vi "1_VNA_direct_spectrum_field_sweep_CURRENT_(2D_PNA_m_Field_Direct_spec_RHUL).vi"() -> ()   [LabVIEW 2013]
uses:
  <vilib>/Analysis/baseanly.llb/Mean (DBL).vi
  <vilib>/Analysis/NI_AALBase.lvlib
panel:
  in  "?":enum32{"Magnetic Field", "Cycle wait"}(tab)
  in  "I_start (mA)":dbl=-10.0 format="%#.3f"
  in  "I_end(mA)":dbl=6953330000.0 caption="Center Freq (Hz):" format="%#.6p"
  in  "n_points":i32=1000
  in  "Current":bool
  out "I current":dbl=3.2196
  in  "Cycle delay (s)":dbl
  in  "First step delay (s)":dbl
  in  "?":enum32{"VNA"}(tab)
  out "Numeric":i32
  in  "No averages":i32=3 caption="Delay Time (s)"
  in  "Background remove":bool
  in  "?":enum32{"VNA"}(tab)
  in  "VNA Power dBm":dbl=-30.0 caption="VNA Power (dBm)" format="%#.3f"
  in  "Center Freq (Hz)":dbl=9000000000.0 caption="Center Freq (Hz):" format="%#.6p"
  in  "Span Freq:":dbl=14000000000.0 caption="Span Freq (Hz)" format="%#.3p"
  in  "Bandwidth:":dbl=10.0 caption="Bandwidth (1 to 1e6 Hz)" format="%#.3f"
  in  "Points:":i32=201 caption="Points"
  out "Phase (now)":dbl[](graph)
  out "Amplitude (now)":dbl[](graph)
  in  "Phase delay (ns)":dbl=53.6 format="%#_8g"
  in  "Offset (rad)":dbl
  out "Phase Background Corrected":dbl[][](graph)
  out "Amplitude Background Corrected":dbl[][](graph)
  out "Phase Raw":dbl[][](graph)
  out "Amplitude Raw":dbl[][](graph)
  out "XY Graph":cluster{dbl[], dbl[]}(graph)
  out "Temp_start":dbl=2.0 format="%#_13g"
  out "Temp_end":dbl=16.0 format="%#_13g"
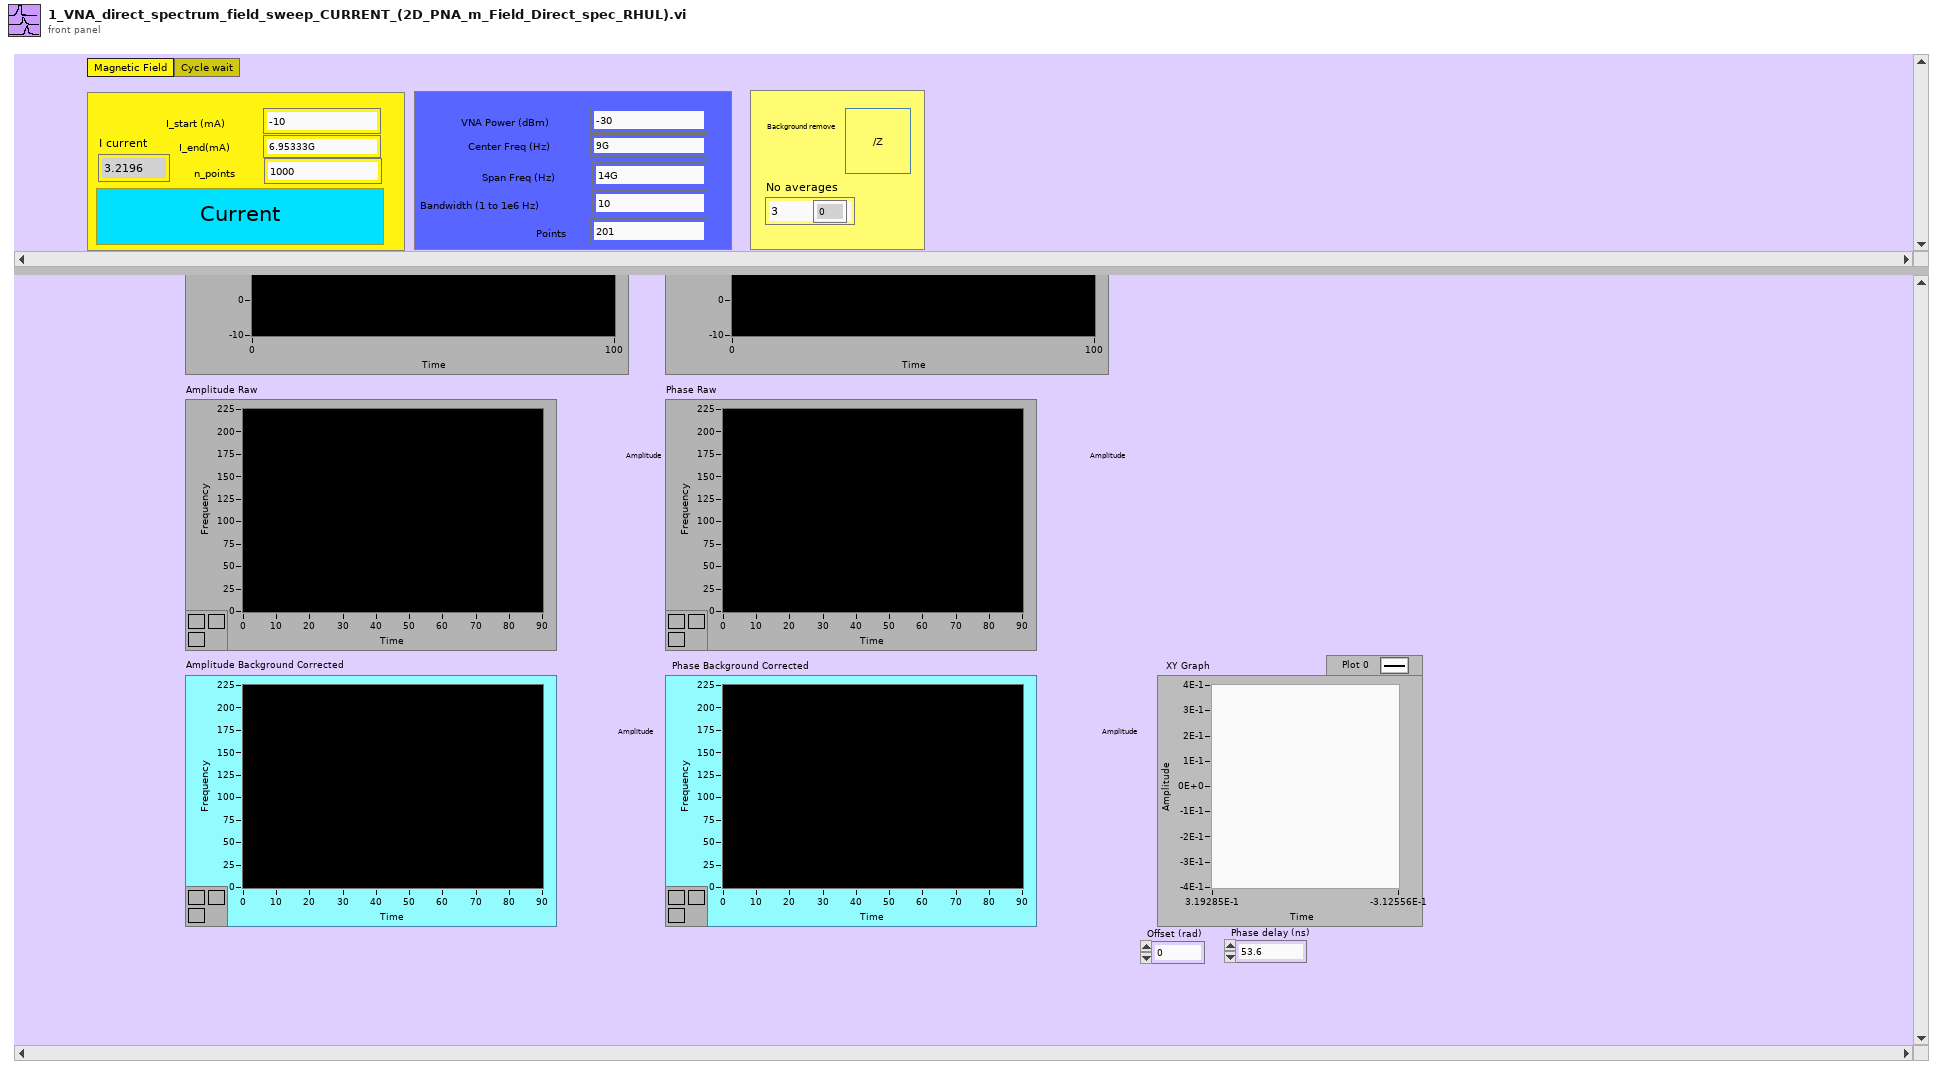
[diagram p1: front panel]
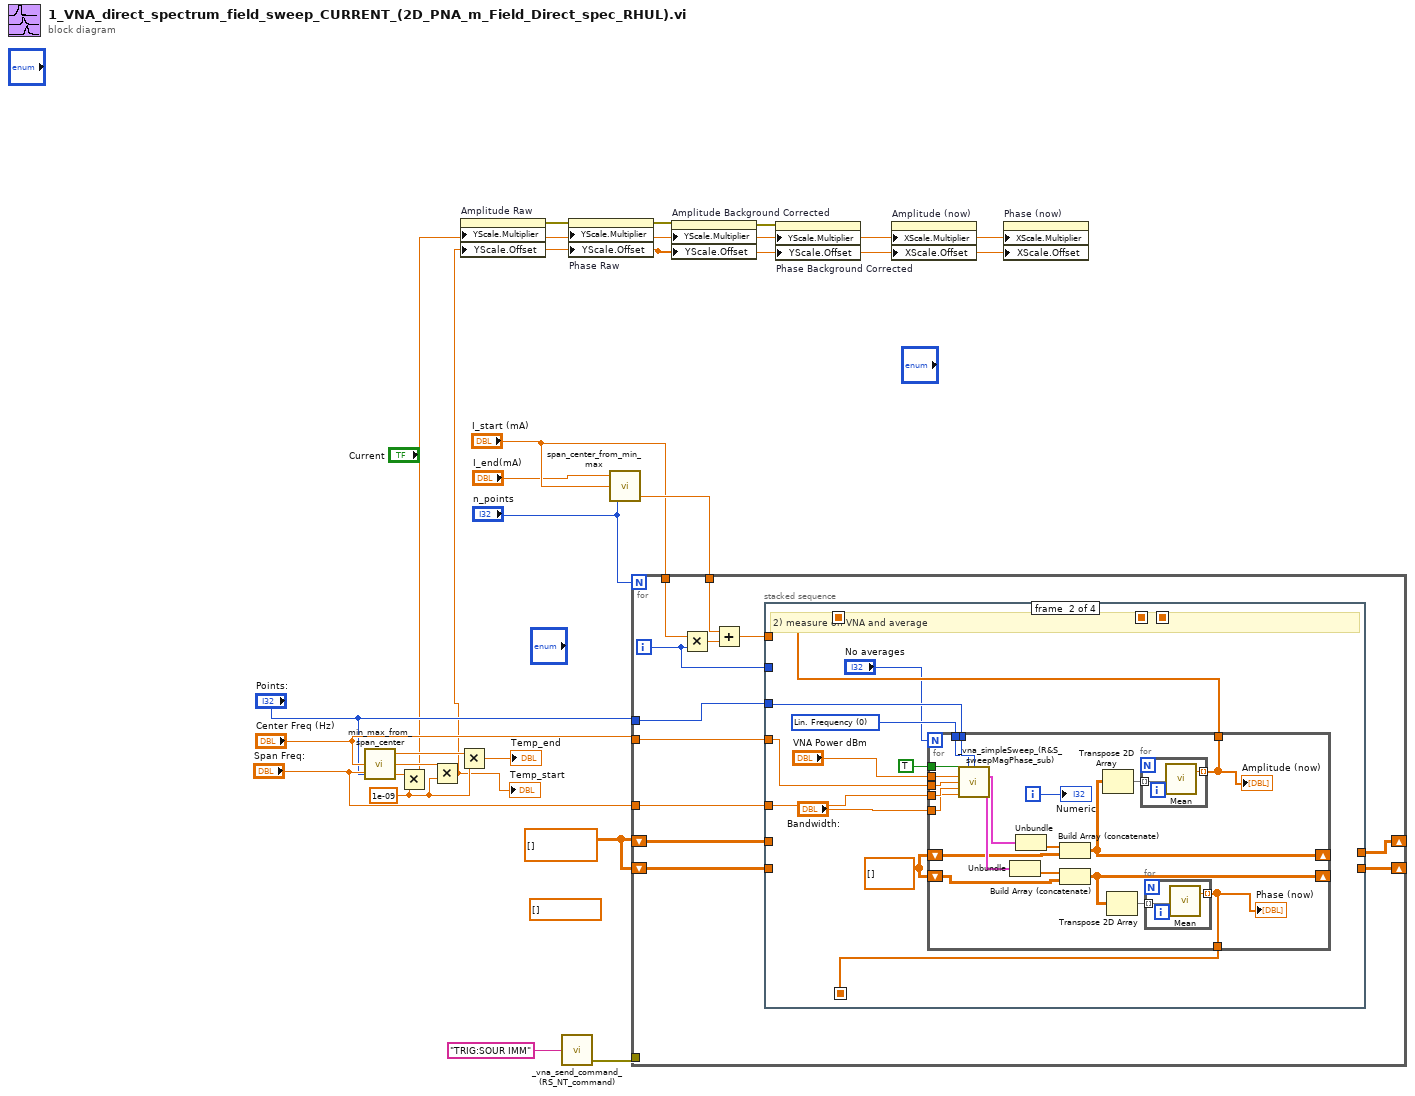
[diagram p0: block diagram]
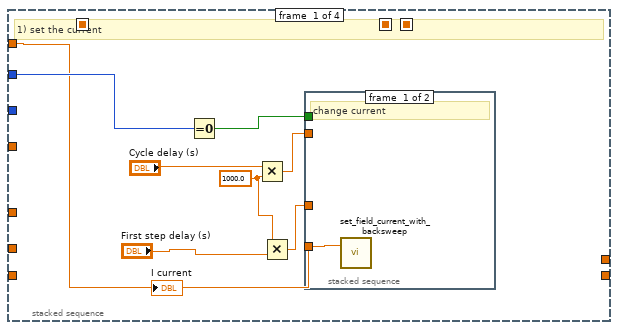
[diagram p2: hidden frame]
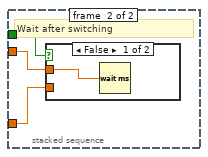
[diagram p3: hidden frame]
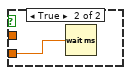
[diagram p4: hidden frame]
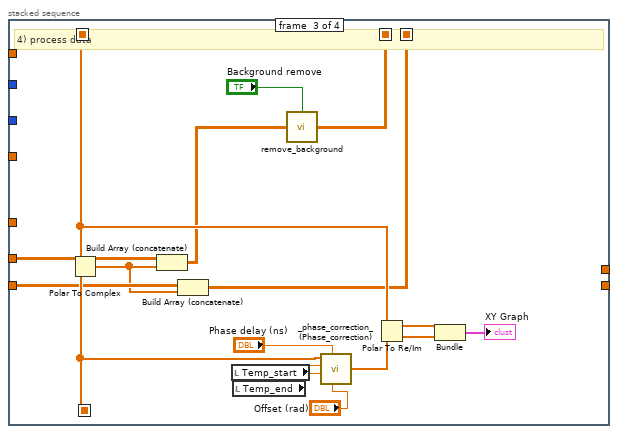
[diagram p5: hidden frame]
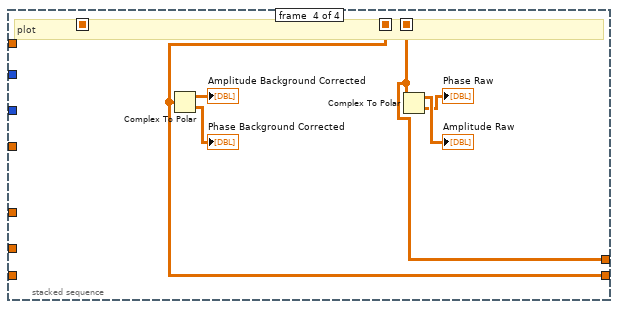
[diagram p6: hidden frame]
diagram:
  (unwired) dbl[] []
  w10 = cdb[][] [] ("Array")
  w13 = 1e-09
  n1 = call "min_max_from_span_center.vi"("No Points"="Points:", "Mid Point"="Center Freq (Hz)", "Span"="Span Freq:") -> ("Step"=w15:dbl, "Start"=w14:dbl, "End"=w18:dbl)
  n2 = Multiply(x=w15, y=w13) -> (x*y=w6:dbl)
  n3 = Multiply(x=w14, y=w13) -> (x*y=w5:dbl)
  "Temp_start" <- w5
  n4 = Multiply(x=w18, y=w13) -> (x*y=→"Temp_end":dbl)
  n5 = property on="Amplitude Raw" class="IntGraph (strict)"("YScale.Multiplier"=w6, "YScale.Offset"=w5) -> (error out=w9:errorcluster)  [unwired: 2 in, 1 out]
  n6 = call "_vna_send_command_(RS_NT_command).vi"("Comand"="TRIG:SOUR IMM") -> ("error out"=w19:errorcluster)  [unwired: 4 in]
  n7 = property on="Phase Raw" class="IntGraph (strict)"(error in=w9, "YScale.Multiplier"=w6, "YScale.Offset"=w5) -> (error out=w7:errorcluster)  [unwired: 1 in, 1 out]
  n8 = call "span_center_from_min_max.vi"("No Points"="n_points", "Begin"="I_start (mA)", "End"="I_end(mA)") -> ("Step"=w4:dbl)  [unwired: 2 out]
  n9 = for {
    N: "n_points" -> [_]
    tunnel: "Center Freq (Hz)" -> [w32]
    tunnel: "Span Freq:" -> [w31]
    tunnel: "Points:" -> [w30]
    tunnel: w19 -> [_]
    shift-right: [w21] -> _
    shift-left: w10 -> [w29]
    shift-right: [w22] -> _
    shift-left: w10 -> [w28]
    tunnel: "I_start (mA)" -> [w27]
    tunnel: w4 -> [w25]
    i -> [w23]
    n10 = Multiply(x=w27, y=w23) -> (x*y=w26:dbl)
    n11 = Add(x=w25, y=w26) -> (x+y=w24:dbl)
    n12 = stacked-sequence {
      seq-local: [_ w49 _ _] -> [_ _ w94 _]
      seq-local: [_ w48 _ _] -> [_ _ w87 _]
      seq-local: [_ _ w82 _] -> [_ _ _ w100]
      seq-local: [_ _ w83 _] -> [_ _ _ w99]
      tunnel: w32 -> [_ w51 _ _]
      tunnel: w31 -> [_ w56 _ _]
      tunnel: w30 -> [_ w57 _ _]
      tunnel: w29 -> [_ _ w93 _]
      tunnel: w28 -> [_ _ w86 _]
      tunnel: w24 -> [w33 _ _ _]
      tunnel: w23 -> [w36 _ _ _]
      tunnel: [_ _ _ w100] -> w22
      tunnel: [_ _ _ w99] -> w21
      frame #0 {
        w37 = 1000.0 ("y")
        # "1) set the current"
        n13 = Equal To 0?(x=w36) -> (x = 0?=w38:bool)
        n14 = Multiply(x="Cycle delay (s)", y=w37) -> (x*y=w39:dbl)
        n15 = Multiply(x=w37, y="First step delay (s)") -> (x*y=w40:dbl)
        n16 = stacked-sequence {
          tunnel: w33 -> [w41 _]
          tunnel: w38 -> [_ w44]
          tunnel: w40 -> [_ w43]
          tunnel: w39 -> [_ w42]
          frame #0 {
            # "change current"
            n17 = call "set_field_current_with_backsweep.vi"("I mA"=w41) -> ()  [unwired: 2 in, 1 out]
          }
          frame #1 {
            # "Wait after switching"
            n18 = case shown="False" w44 {
              tunnel: w43 -> [_ w46]
              tunnel: w42 -> [w45 _]
              frame False {
                n19 = Wait (ms)(milliseconds to wait=w45) -> ()  [unwired: 1 out]
              }
              frame True {
                n20 = Wait (ms)(milliseconds to wait=w46) -> ()  [unwired: 1 out]
              }
            }
          }
        }
        "I current" <- w33
      }
      frame #1 {
        w50 = dbl[][] []
        w55 = 0 items=["Lin. Frequency", "Log. Frequency", "Segmented Frequency", "Power", "Time", "CW Mode"] ("Sweep Type")
        # "2) measure on VNA and average"
        n21 = for {
          N: "No averages" -> [_]
          tunnel: w57 -> [w75]
          tunnel: w56 -> [w74]
          tunnel: w55 -> [w73]
          tunnel: TRUE ("Boolean") -> [w72]
          tunnel: "VNA Power dBm" -> [w71]
          tunnel: "Bandwidth:" -> [w70]
          tunnel: w51 -> [w69]
          shift-right: [w64] -> _
          shift-left: w50 -> [w66]
          shift-right: [w61] -> _
          shift-left: w50 -> [w65]
          tunnel: [w60] -> w49
          tunnel: [w59] -> w48
          i -> [w58]
          n22 = call "_vna_simpleSweep_(R&S_sweepMagPhase_sub).vi"("Boolean"=w72, "Sweep Type"=w73, "Points:"=w75, "Power dBm"=w71, "Center Freq:"=w69, "Span Freq:"=w74, "Bandwidth:"=w70) -> ("Lin Mag"=w77:cluster{dbl[], dbl[]}, "Phase"=w76:cluster{dbl[], dbl[]})  [unwired: 7 in]
          n23 = Unbundle(w76) -> (w68:dbl[])  [unwired: 1 out]
          n24 = Unbundle(w77) -> (w67:dbl[])  [unwired: 1 out]
          n25 = Build Array (concatenate)(w67, w66) -> (w64:dbl[][])
          n26 = Build Array (concatenate)(w68, w65) -> (w61:dbl[][])
          n27 = Transpose 2D Array(2D array=w64) -> (transposed array=w63:dbl[][])
          n28 = Transpose 2D Array(2D array=w61) -> (transposed array=w62:dbl[][])
          n29 = for {
            tunnel: w63 -> [w81] mode=indexing
            tunnel: [w80] -> w60 mode=indexing
            n30 = call-poly <vilib>:"Mean.vi"("X"=w81) -> ("mean"=w80:dbl)  [unwired: 1 out]
          }
          "Amplitude (now)" <- w60
          n31 = for {
            tunnel: w62 -> [w79] mode=indexing
            tunnel: [w78] -> w59 mode=indexing
            n32 = call-poly <vilib>:"Mean.vi"("X"=w79) -> ("mean"=w78:dbl)  [unwired: 1 out]
          }
          "Phase (now)" <- w59
          "Numeric" <- w58
        }
      }
      frame #2 {
        # "4) process data"
        n33 = Polar To Complex(1:w87, 2:w94) -> (0:w85:cdb[])
        n34 = Build Array (concatenate)(w93, w85) -> (w92:cdb[][])
        n35 = Build Array (concatenate)(w86, w85) -> (w83:cdb[][])
        n36 = local read "Temp_start"() -> (w89:dbl)
        n37 = local read "Temp_end"() -> (w90:dbl)
        n38 = call "remove_background.vi"("Array in"=w92, "Boolean"="Background remove") -> ("Array out"=w82:cdb[][])
        n39 = call "_phase_correction_(Phase_correction).vi"("offset"="Offset (rad)", "Delay (ns)"="Phase delay (ns)", "f1 (GHz)"=w90, "f0 (GHz)"=w89, "Phase in"=w87) -> ("Phase out"=w95:dbl[])  [unwired: 4 in]
        n40 = Polar To Re/Im(2:w95, 3:w94) -> (0:w97:dbl[], 1:w98:dbl[])
        n41 = Bundle(w98, w97) -> (→"XY Graph":cluster{dbl[], dbl[]})  [unwired: 1 in]
      }
      frame #3 {
        # "plot"
        n42 = Complex To Polar(r * e^(i*theta)=w100) -> (r=→"Amplitude Background Corrected":dbl[][], theta=→"Phase Background Corrected":dbl[][])
        n43 = Complex To Polar(r * e^(i*theta)=w99) -> (r=→"Amplitude Raw":dbl[][], theta=→"Phase Raw":dbl[][])
      }
    }
  }
  n44 = property on="Amplitude Background Corrected" class="IntGraph (strict)"(error in=w7, "YScale.Multiplier"=w6, "YScale.Offset"=w5) -> (error out=w8:errorcluster)  [unwired: 1 in, 1 out]
  n45 = property on="Phase Background Corrected" class="IntGraph (strict)"(error in=w8, "YScale.Multiplier"=w6, "YScale.Offset"=w5) -> ()  [unwired: 1 in, 2 out]
  n46 = property on="Amplitude (now)" class="WFChart (strict)"("XScale.Multiplier"=w6, "XScale.Offset"=w5) -> ()  [unwired: 2 in, 2 out]
  n47 = property on="Phase (now)" class="WFChart (strict)"("XScale.Multiplier"=w6, "XScale.Offset"=w5) -> ()  [unwired: 2 in, 2 out]
